vi "GetPythonFunction.vi"(5 "function name":string, 6 "error in":errorcluster, 9 "PythonConverter_BD in":refnum<class "PyConvBD.lvclass">) -> (0 "error out":errorcluster, 3 "PythonConverter_BD out":refnum<class "PyConvBD.lvclass">, 4 "Python function":refnum<class "PythonFunction.lvclass">)   [LabVIEW 2014, in "PyConvBD.lvclass"]
uses:
  PyConvBD.lvclass
  Parsing/Classes/PythonFunction/PythonFunction.lvclass
  PyConvBD.lvclass/PyConvBD.ctl
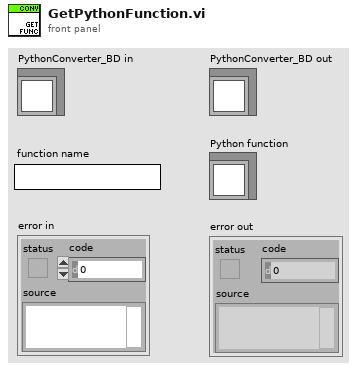
[diagram p1: front panel]
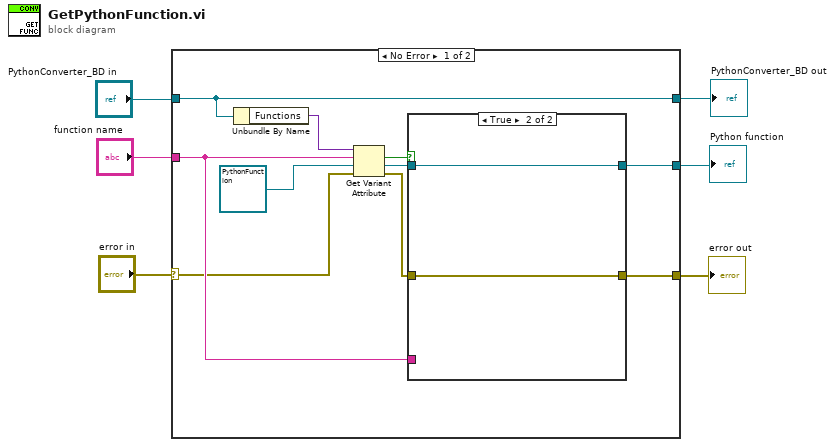
[diagram p0: block diagram]
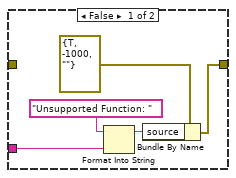
[diagram p2: hidden frame]
diagram:
  n1 = case shown="No Error" "error in" {
    selector: "error in" -> [w8 w24]
    tunnel: "PythonConverter_BD in" -> [w7 w25]
    tunnel: [w12 _] -> w6
    tunnel: "function name" -> [w10 _]
    tunnel: [w9 w24] -> w4
    tunnel: [w7 w25] -> w2
    frame No Error {
      n2 = Unbundle By Name(w7) -> ("Functions"=w16:variant)
      n3 = Get Variant Attribute(Variant=w16, name=w10, default value (empty Variant)=refnum<class "PythonFunction.lvclass"> refnum ("Python function"), error in=w8) -> (found=w15:bool, value=w13:refnum<class "PythonFunction.lvclass">, error out=w14:errorcluster)  [unwired: 1 out]
      n4 = case shown="True" w15 {
        tunnel: w14 -> [_ w23]
        tunnel: [w18 w23] -> w9
        tunnel: w13 -> [_ w22]
        tunnel: [_ w22] -> w12
        tunnel: w10 -> [w21 _]
        frame False {
          n5 = Format Into String(initial string="Unsupported Function: " ("source"), w21) -> (resulting string=w17:string)  [unwired: 2 in, 1 out]
          n6 = Bundle By Name(cluster=errorcluster {"status"=TRUE, "code"=-1000, "source"=""} ("error out"), "source"=w17) -> (w18:errorcluster)
        }
        frame True {
        }
      }
    }
    frame Error {
    }
  }
  "error out" <- w4
  "PythonConverter_BD out" <- w2
  "Python function" <- w6
